vi "Eagle_RT Scanner Timing Tests.vi"() -> ()   [LabVIEW 2015]
uses:
  <vilib>/Platform/TimedLoop/XDataNode/timing_clust.ctl
  <vilib>/Platform/TimedLoop/XDataNode/nitl_modes.ctl
  <vilib>/Platform/TimedLoop/XDataNode/wakeup.ctl
  <vilib>/FPGAPlugInAG/cRIO-9030/niLvFpga_Open_cRIO-9030.vi
  <vilib>/rvi/interface/common/dynamic/niFpgaDynamicAddResources.vi
  <vilib>/FPGAPlugInAG/Dynamic/niLvFpga_Run_Dynamic.vi
  <vilib>/Utility/error.llb/Error Cluster From Error Code.vi
  <vilib>/rvi/errors/niLvFpgaAdjustHostInterfaceError.vi
  <vilib>/rvi/interface/nirviOpenFPGA/nirviOpenFPGA.xnode
  FPGA Bitfiles/BELKINEAGLEGUI_FPGATarget_EagleFPGAScanner_juOkZGXIgM0.lvbitx
  Eagle_FPGA Scanner Control.vi
  <vilib>/rvi/interface/nirviMethod/nirviMethod.xnode
  <vilib>/rvi/interface/nirviReadWriteControl/nirviReadWriteControl.xnode
  <vilib>/Platform/TimedLoop/XDataNode/XDataNode.xnode
  <vilib>/Platform/TimedLoop/XDataNode/XDNodeRunTimeDep.lvlib
  NiFpgaLv.dll
  <vilib>/rvi/interface/Simulation/niFpgaSimulationCallBeginRW.vi
panel:
  out "Array 4":i32[](array[numeric])
  out "x-y":u32
  out "Array 3":fxp<+/-,20,5>[](array[numeric])
  out "Array 2":fxp<+/-,20,5>[](array[numeric])
  in  "Count(uSec)":u32
  out "Array":fxp<+/-,20,5>[](array[numeric])
  # "122"
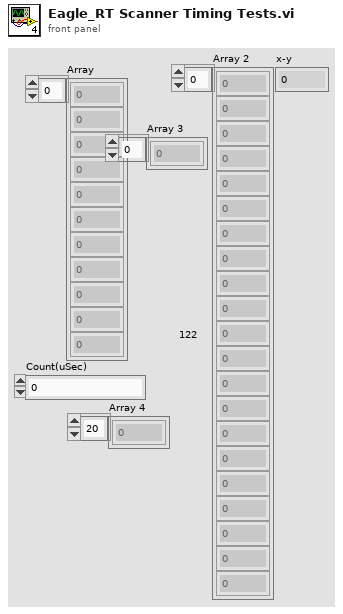
[diagram p1: front panel]
types:
  T1 = typedef "XDNodeRunTimeDep.lvlib/timing_clust.ctl" = cluster{"Expected End [f-1]":u64, "Actual End [f-1]":u64, "Finished Late? [f-1]":bool, "Expected End [i-1]":u64, "Actual End [i-1]":u64, "Finished Late? [i-1]":bool, "Expected Start [i]":u64, "Actual Start [i]":u64, "Expected Start [f]":u64, "Actual Start [f]":u64, "Source Name":string, "Structure Name":string, "Period":i64, "Deadline":i64, "Offset":i64, "Start":i64, "Priority":i32, "Timeout":i32, "Mode":T2, "Wakeup Reason":T3, "Error":errorcluster, "Source Type":string, "Secondary Source Type":string, "Global End Time":u64, "Global Start Time":u64, "Frame Duration":u64, "Iteration Duration":u64, "Assigned CPU":i32, "I/O Scan Engine Mode":u32}
  T2 = typedef "XDNodeRunTimeDep.lvlib/nitl_modes.ctl" = enum32{"No Change", "Process missed periods, maintain original phase", "Discard missed periods, maintain original phase", "Process missed periods, ignore original phase", "Discard missed periods, ignore original phase"}
  T3 = typedef "XDNodeRunTimeDep.lvlib/wakeup.ctl" = enum32{"Normal", "Aborted", "Asynchronous wakeup", "Timing source error", "Timed loop error", "Timeout"}
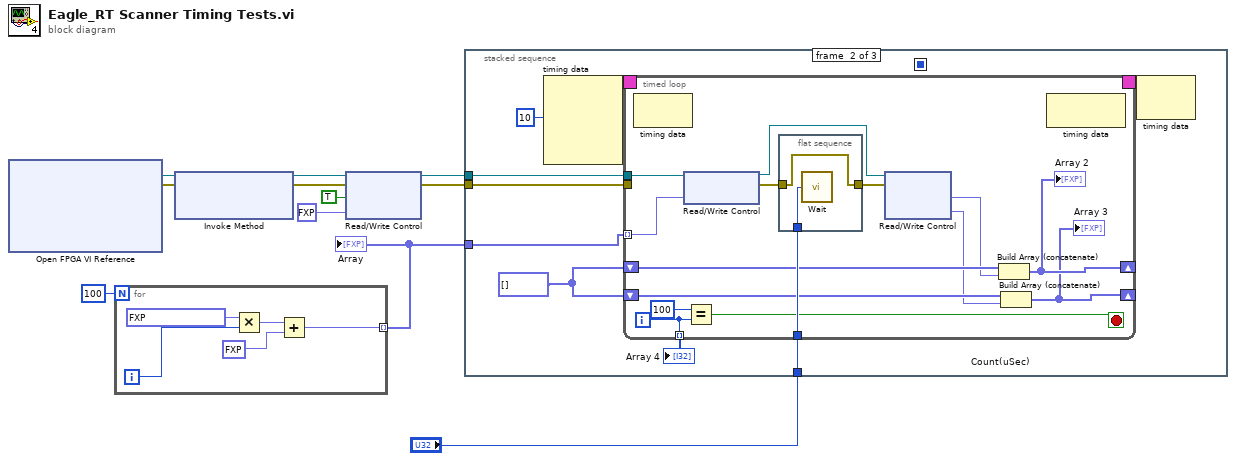
[diagram p0: block diagram]
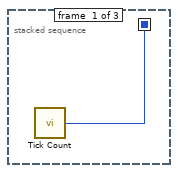
[diagram p2: hidden frame]
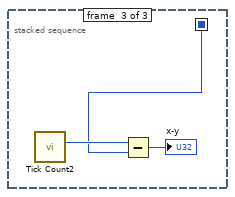
[diagram p3: hidden frame]
diagram:
  n1 = xnode "Open FPGA VI Reference"() -> ("FPGA VI Reference Out"=w11:refnum<k20>, "error out"=w8:errorcluster)  [unwired: 2 in]
  n2 = for {
    N: 100 -> [_]
    tunnel: [w12] -> w1 mode=indexing
    i -> [w15]
    n3 = Multiply(x=fxp<+/-,20,5> 0.20001220703125, y=w15) -> (x*y=w14:fxp<+/-,52,37>)
    n4 = Add(x=w14, y=fxp<+/-,20,5> -10.0 ("x")) -> (x+y=w12:fxp<+/-,52,37>)
  }
  "Array" <- w1
  n5 = xnode "Invoke Method"("FPGA VI Reference In"=w11, "error in"=w8) -> ("FPGA VI Reference Out"=w10:refnum<k20>, "error out"=w9:errorcluster)  [unwired: 1 in]
  n6 = xnode "Read/Write Control"("FPGA VI Reference In"=w10, "error in"=w9, "Manual"=TRUE, "Manual VY"=fxp<+/-,20,5> 0.0) -> ("FPGA VI Reference Out"=w4:refnum<k20>, "error out"=w6:errorcluster)
  n7 = stacked-sequence {
    seq-local: [w17 _ _] -> [_ _ w51]
    tunnel: w6 -> [_ w23 _]
    tunnel: w4 -> [_ w22 _]
    tunnel: w1 -> [_ w21 _]
    tunnel: "Count(uSec)" -> [_ w20 _]
    frame #0 {
      n8 = call "Tick Count"() -> ("Tick Count(uSec)"=w17:u32)
    }
    frame #1 {
      w19 = fxp<+/-,20,5>[] [] ("Array 2")
      n9 = node-c288(i64 10 ("Period")) -> (w26:T1)  [unwired: 3 in]
      n10 = timed-loop {
        timing: w26 -> [_]
        timing-out: [_] -> w25
        tunnel: w23 -> [_]
        tunnel: w22 -> [w41]
        tunnel: w21 -> [w40] mode=indexing
        tunnel: w20 -> [w38]
        shift-right: [w31] -> _
        shift-left: w19 -> [w35]
        shift-right: [w30] -> _
        shift-left: w19 -> [w33]
        tunnel: [w27] -> w18 mode=indexing
        i -> [w27]
        stop <- w28 stop-if-true
        n11 = node-c288() -> ()  [unwired: 1 in, 1 out]
        n12 = xnode "Read/Write Control"("FPGA VI Reference In"=w41, "Manual VX"=w40) -> ("FPGA VI Reference Out"=w37:refnum<k20>, "error out"=w39:errorcluster)  [unwired: 1 in]
        n13 = Equal?(x=100, y=w27) -> (x = y?=w28:bool)
        n14 = flat-sequence {
          tunnel: w39 -> [w42]
          tunnel: w38 -> [w43]
          tunnel: [w42] -> w36
          frame #0 {
            n15 = call "Wait"("Count(uSec)"=w43) -> ()  [unwired: 1 out]
          }
        }
        n16 = xnode "Read/Write Control"("FPGA VI Reference In"=w37, "error in"=w36) -> ("X READ 2"=w34:fxp<+/-,20,5>, "Y READ 2"=w32:fxp<+/-,20,5>)  [unwired: 2 out]
        n17 = Build Array (concatenate)(w35, w34) -> (w31:fxp<+/-,20,5>[])
        "Array 2" <- w31
        n18 = Build Array (concatenate)(w33, w32) -> (w30:fxp<+/-,20,5>[])
        "Array 3" <- w30
        n19 = node-c288() -> ()  [unwired: 1 in, 1 out]
      }
      "Array 4" <- w18
      n20 = node-c288(w25) -> ()  [unwired: 1 out]
    }
    frame #2 {
      n21 = call "Tick Count2"() -> ("Tick Count(uSec)"=w52:u32)
      n22 = Subtract(x=w52, y=w51) -> (x-y=→"x-y":u32)
    }
  }
